vi "7.3.1_참조.vi"(0 "비활성화":T1(ring), 1 "디스플레이 스타일":u32, 2 "Str 참조 번호":refnum<vi>, 3 "Bool 참조 번호":refnum<vi>) -> ()   [LabVIEW 2018]
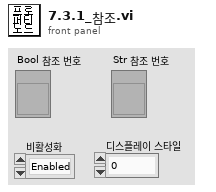
[diagram p1: front panel]
types:
  T1 = enum8{"Enabled", "Disabled", "Disabled and Grayed Out"}
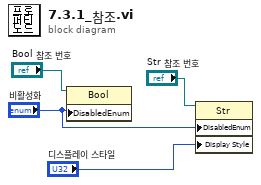
[diagram p0: block diagram]
diagram:
  n1 = property class="Bool"(reference="Bool 참조 번호", "DisabledEnum"="비활성화") -> ()  [unwired: 1 in, 2 out]
  n2 = property class="Str"(reference="Str 참조 번호", "DisabledEnum"="비활성화", "Display Style"="디스플레이 스타일") -> ()  [unwired: 1 in, 2 out]
